vi "Do.vi"(8 "error in (no error)":errorcluster, 10 "Parent Actor":refnum<class "Parent Actor.lvclass">, 11 "Turn On in":refnum<class "Turn On.lvclass">) -> (0 "error out":errorcluster, 2 "Parent Actor out":refnum<class "Parent Actor.lvclass">, 3 "Turn On out":refnum<class "Turn On.lvclass">)   [LabVIEW 2015, in "Turn On.lvclass"]
uses:
  Turn On.lvclass
  State/Parent Actor.lvclass
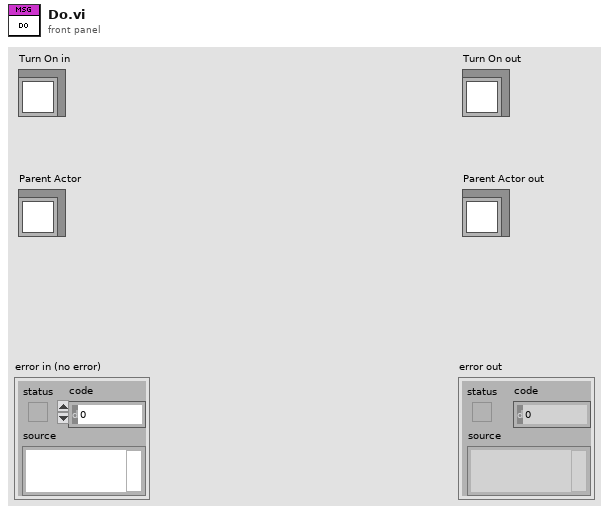
[diagram p1: front panel]
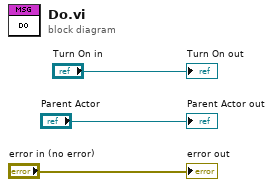
[diagram p0: block diagram]
diagram:
  "error out" <- "error in (no error)"
  "Turn On out" <- "Turn On in"
  "Parent Actor out" <- "Parent Actor"
